vi "Galvo_String.vi"(0 "xStart":dbl[](array[numeric]), 1 "xEnd":dbl[](array[numeric]), 2 "#Ascans":i32, 3 "yStart":dbl[](array[numeric]), 4 "yEnd":dbl[](array[numeric]), 5 "#GalvoReposition":i32, 8 "#Silent Samples":i32) -> (6 "xGalvo":dbl[](graph), 9 "yGalvo":dbl[](graph))   [LabVIEW 2017]
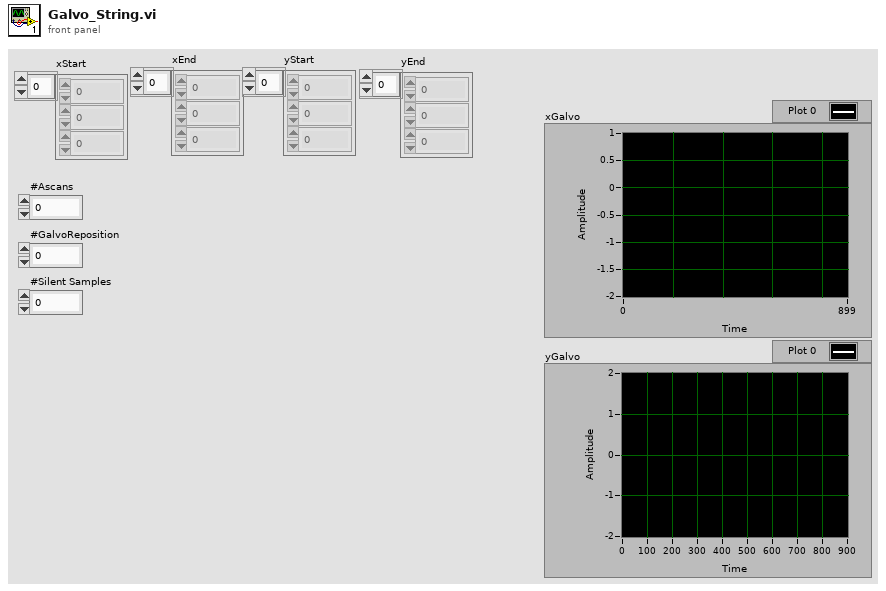
[diagram p1: front panel]
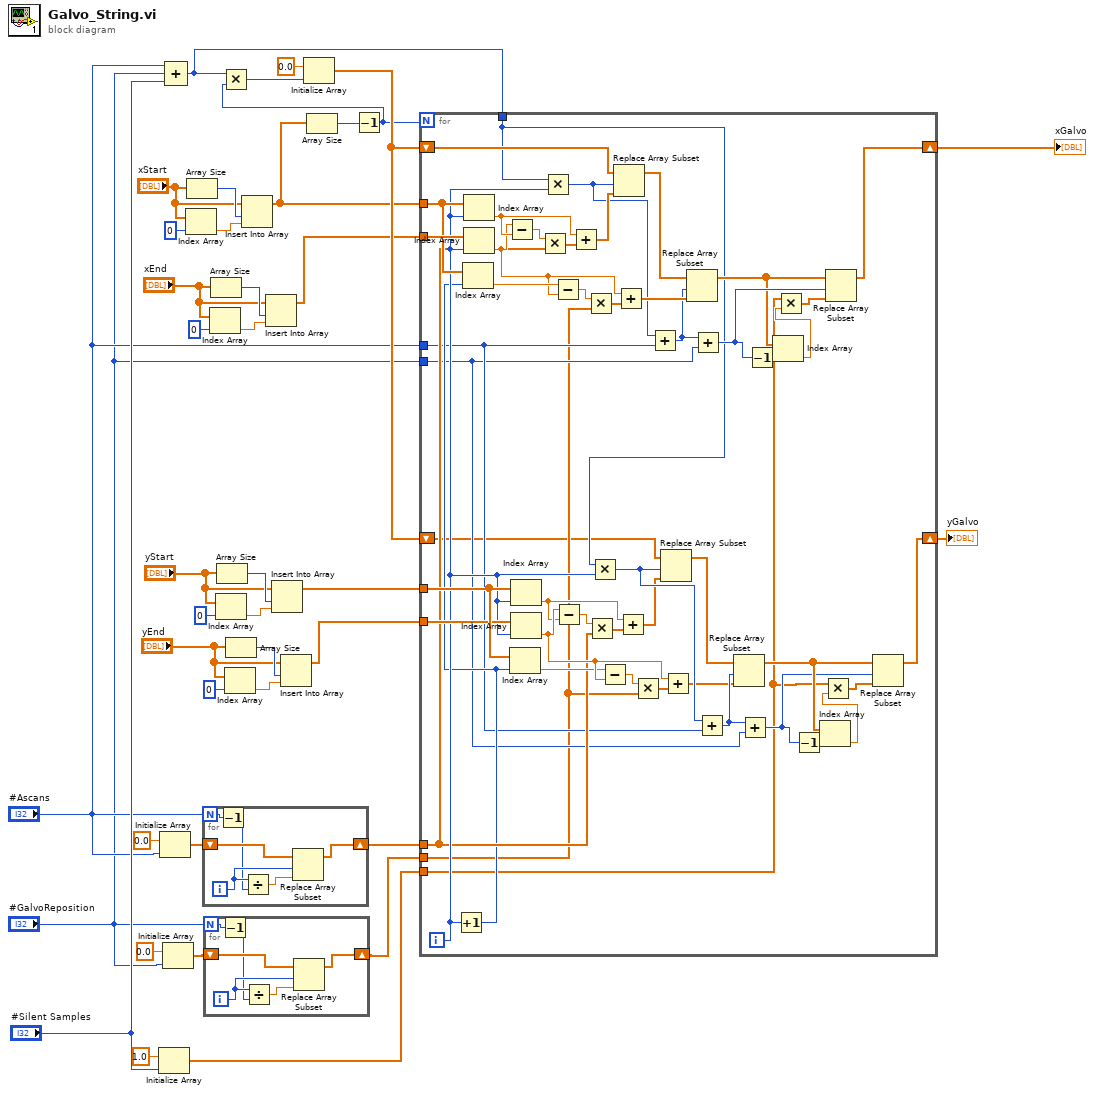
[diagram p0: block diagram]
diagram:
  n1 = Initialize Array(1.0 ("element"), "#Silent Samples") -> (w24:dbl[])
  n2 = Initialize Array(0.0 ("element"), "#Ascans") -> (w38:dbl[])
  n3 = Initialize Array(0.0 ("element"), "#GalvoReposition") -> (w34:dbl[])
  n4 = Compound Arithmetic op=ADD("#Ascans", "#GalvoReposition", "#Silent Samples") -> (w27:i32)
  n5 = Index Array(array="xStart", index=0) -> (element=w19:dbl)
  n6 = Array Size(array="xStart") -> (size(s)=w21:i32)
  n7 = for {
    N: "#Ascans" -> [w42]
    shift-right: [w44] -> w35
    shift-left: w38 -> [w45]
    i -> [w43]
    n8 = Decrement(x=w42) -> (x-1=w40:i32)
    n9 = Divide(x=w43, y=w40) -> (x/y=w41:dbl)
    n10 = Replace Array Subset(array=w45, new element=w41, index=w43) -> (w44:dbl[])
  }
  n11 = for {
    N: "#GalvoReposition" -> [w48]
    shift-right: [w50] -> w33
    shift-left: w34 -> [w51]
    i -> [w49]
    n12 = Decrement(x=w48) -> (x-1=w46:i32)
    n13 = Divide(x=w49, y=w46) -> (x/y=w47:dbl)
    n14 = Replace Array Subset(array=w51, new element=w47, index=w49) -> (w50:dbl[])
  }
  n15 = Index Array(array="xEnd", index=0) -> (element=w14:dbl)
  n16 = Array Size(array="xEnd") -> (size(s)=w16:i32)
  n17 = Index Array(array="yStart", index=0) -> (element=w9:dbl)
  n18 = Array Size(array="yStart") -> (size(s)=w11:i32)
  n19 = Index Array(array="yEnd", index=0) -> (element=w4:dbl)
  n20 = Array Size(array="yEnd") -> (size(s)=w6:i32)
  n21 = Insert Into Array(array="xStart", index=w21, new element=w19) -> (w17:dbl[])
  n22 = Insert Into Array(array="xEnd", index=w16, new element=w14) -> (w13:dbl[])
  n23 = Insert Into Array(array="yStart", index=w11, new element=w9) -> (w7:dbl[])
  n24 = Insert Into Array(array="yEnd", index=w6, new element=w4) -> (w2:dbl[])
  n25 = Array Size(array=w17) -> (size(s)=w31:i32)
  n26 = Decrement(x=w31) -> (x-1=w1:i32)
  n27 = Multiply(x=w27, y=w1) -> (x*y=w30:i32)
  n28 = Initialize Array(0.0 ("element"), w30) -> (w28:dbl[])
  n29 = for {
    N: w1 -> [_]
    tunnel: w17 -> [w95]
    tunnel: w13 -> [w101]
    tunnel: w7 -> [w62]
    tunnel: w2 -> [w61]
    tunnel: w35 -> [w59]
    tunnel: w33 -> [w55]
    shift-right: [w81] -> w26
    shift-left: w28 -> [w96]
    shift-right: [w53] -> w22
    shift-left: w28 -> [w52]
    tunnel: w27 -> [w63]
    tunnel: "#Ascans" -> [w57]
    tunnel: w24 -> [w54]
    tunnel: "#GalvoReposition" -> [w56]
    i -> [w60]
    n30 = Increment(x=w60) -> (x+1=w58:i32)
    n31 = Index Array(array=w95, index=w58) -> (element=w93:dbl)
    n32 = Index Array(array=w95, index=w60) -> (element=w98:dbl)
    n33 = Index Array(array=w101, index=w60) -> (element=w92:dbl)
    n34 = Subtract(x=w92, y=w98) -> (x-y=w100:dbl)
    n35 = Index Array(array=w62, index=w58) -> (element=w69:dbl)
    n36 = Index Array(array=w62, index=w60) -> (element=w66:dbl)
    n37 = Index Array(array=w61, index=w60) -> (element=w70:dbl)
    n38 = Multiply(x=w100, y=w59) -> (x*y=w99:dbl[])
    n39 = Multiply(x=w63, y=w60) -> (x*y=w88:i32)
    n40 = Subtract(x=w93, y=w92) -> (x-y=w94:dbl)
    n41 = Subtract(x=w70, y=w66) -> (x-y=w64:dbl)
    n42 = Add(x=w98, y=w99) -> (x+y=w97:dbl[])
    n43 = Multiply(x=w94, y=w55) -> (x*y=w91:dbl[])
    n44 = Multiply(x=w64, y=w59) -> (x*y=w65:dbl[])
    n45 = Multiply(x=w63, y=w60) -> (x*y=w74:i32)
    n46 = Subtract(x=w69, y=w70) -> (x-y=w68:dbl)
    n47 = Replace Array Subset(array=w96, new element=w97, index=w88) -> (w90:dbl[])
    n48 = Add(x=w92, y=w91) -> (x+y=w89:dbl[])
    n49 = Add(x=w66, y=w65) -> (x+y=w67:dbl[])
    n50 = Multiply(x=w68, y=w55) -> (x*y=w71:dbl[])
    n51 = Add(x=w88, y=w57) -> (x+y=w87:i32)
    n52 = Replace Array Subset(array=w52, new element=w67, index=w74) -> (w72:dbl[])
    n53 = Add(x=w70, y=w71) -> (x+y=w73:dbl[])
    n54 = Replace Array Subset(array=w90, new element=w89, index=w87) -> (w82:dbl[])
    n55 = Add(x=w87, y=w56) -> (x+y=w85:i32)
    n56 = Add(x=w74, y=w57) -> (x+y=w75:i32)
    n57 = Replace Array Subset(array=w72, new element=w73, index=w75) -> (w80:dbl[])
    n58 = Add(x=w75, y=w56) -> (x+y=w77:i32)
    n59 = Decrement(x=w85) -> (x-1=w84:i32)
    n60 = Index Array(array=w82, index=w84) -> (element=w83:dbl)
    n61 = Multiply(x=w54, y=w83) -> (x*y=w86:dbl[])
    n62 = Decrement(x=w77) -> (x-1=w78:i32)
    n63 = Index Array(array=w80, index=w78) -> (element=w79:dbl)
    n64 = Multiply(x=w54, y=w79) -> (x*y=w76:dbl[])
    n65 = Replace Array Subset(array=w82, new element=w86, index=w85) -> (w81:dbl[])
    n66 = Replace Array Subset(array=w80, new element=w76, index=w77) -> (w53:dbl[])
  }
  "xGalvo" <- w26
  "yGalvo" <- w22
